vi "frw_array2edf.vi"(6 "channel names":string[](array[string]), 8 "error in":errorcluster, 9 "fs":dbl, 10 "2D array":dbl[][](array[numeric]), 11 "file path":path) -> (0 "error out":errorcluster, 3 "path out":path)   [LabVIEW 2013]
panel:
  out "data_to_write":u16[][](array[numeric])
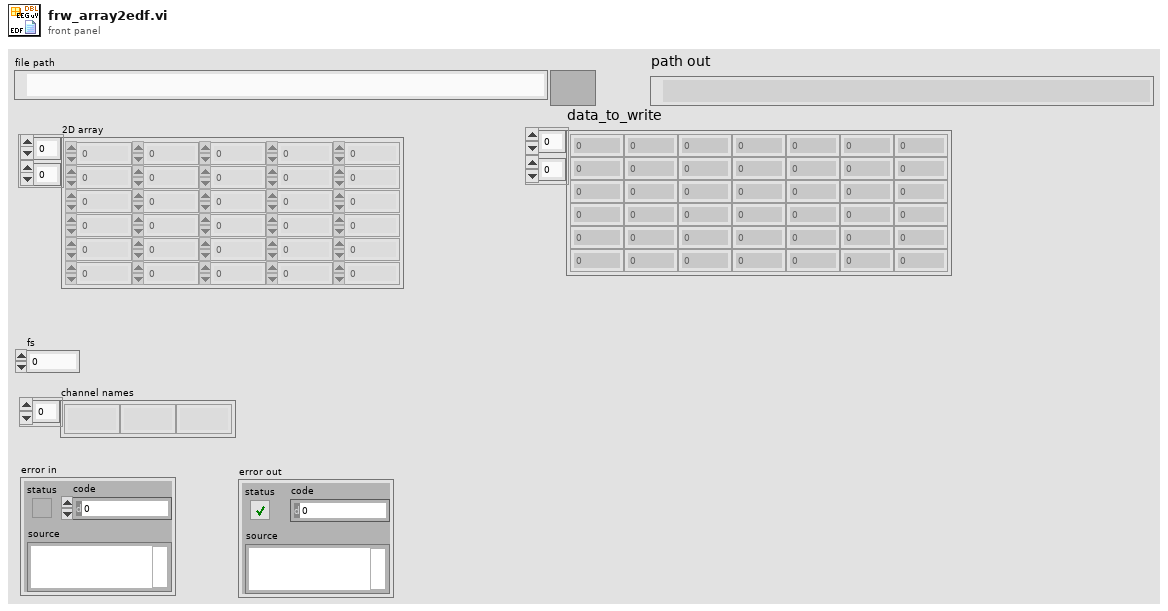
[diagram p1: front panel]
types:
  T1 = enum16{"big-endian, network order", "native, host order", "little-endian"}
  T2 = enum16{"open", "replace", "create", "open or create", "replace or create", "replace or create with confirmation"}
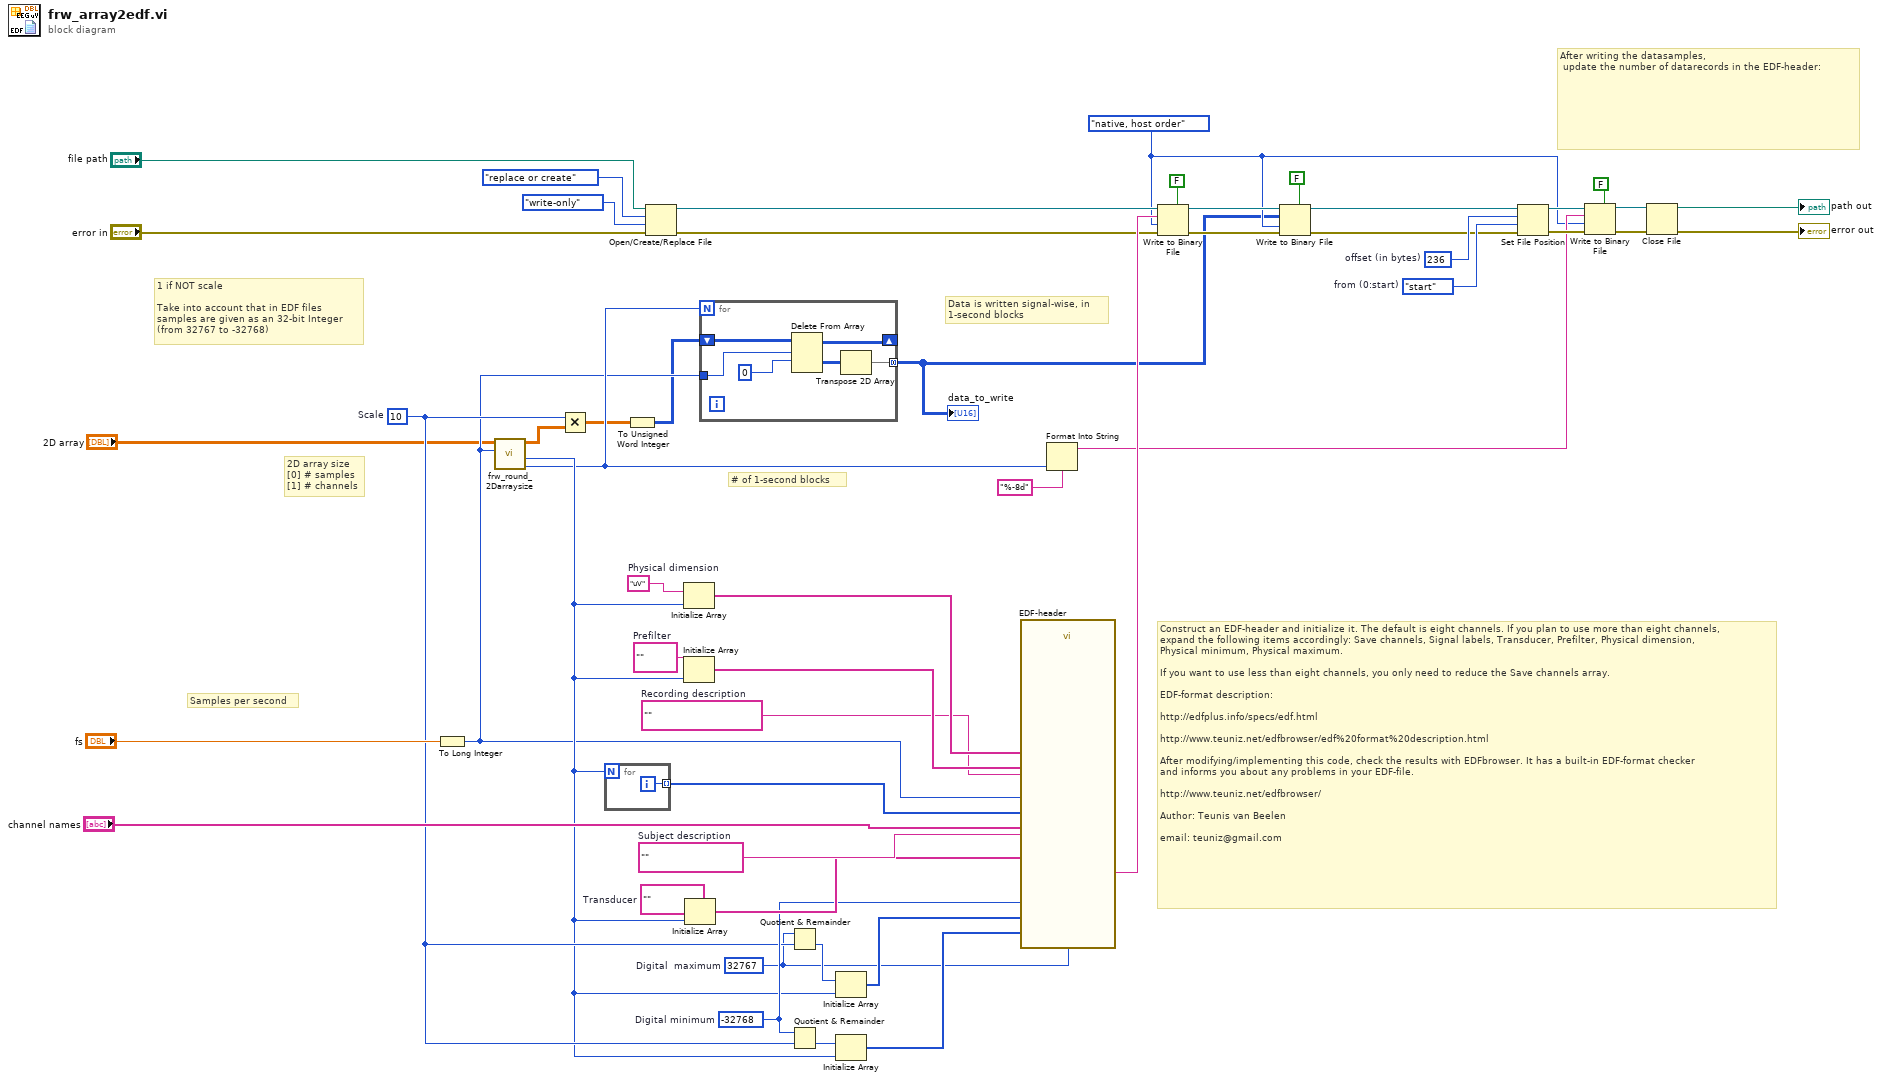
[diagram p0: block diagram]
diagram:
  w15 = 10  # Scale
  w22 = ""  # Transducer
  w23 = ""  # Subject description
  w27 = ""  # Recording description
  w29 = ""  # Prefilter
  w31 = "uV"  # Physical dimension
  w38 = i64 236  # offset (in bytes)
  w39 = enum16{"start", "end", "current"}."start"  # from (0:start)
  w9 = 32767  # Digital  maximum
  w16 = -32768  # Digital minimum
  w12 = T1."native, host order" ("byte order (0:big-endian, network order)")
  # "Data is written signal-wise, in \n1-second blocks"
  # "# of 1-second blocks"
  # "Samples per second"
  # "2D array size\n[0] # samples\n[1] # channels"
  # "1 if NOT scale\n\nTake into account that in EDF files\nsamples are given as an 32-bit Integer\n(from 32767 to -32768)"
  # "After writing the datasamples,\n update the number of datarecords in the EDF-header:"
  # "Construct an EDF-header and initialize it. The default is eight channels. If you plan to use more than eight channels,\nexpand the following items accordingly: Save channels, Signal labels, Transducer, Prefilter, Physical dimension,\nPhysical minimum, Physical maximum.\n\nIf you want to use less than eight channels, you only need to reduce the Save channels array.\n\nEDF-format description:\n\nhttp://edfplus.info/specs/edf.html\n\nhttp://www.teuniz.net/edfbrowser/edf%20format%20description.html\n\nAfter modifying/implementing this code, check the results with EDFbrowser. It has a built-in EDF-format checker\nand informs you about any problems in your EDF-file.\n\nhttp://www.teuniz.net/edfbrowser/\n\nAuthor: Teunis van Beelen\n\nemail: teuniz@gmail.com"
  n1 = To Long Integer(number="fs") -> (32bit integer=w5:i32)
  n2 = call "frw_round_2Darraysize.vi"("block size"=w5, "array in"="2D array") -> ("nBlocks"=w8:i32, "nCol"=w10:i32, "array out"=w7:dbl[][])  [unwired: 6 in, 1 out]
  n3 = Multiply(x=w15, y=w7) -> (x*y=w6:dbl[][])
  n4 = for {
    N: w10 -> [_]
    tunnel: [w52] -> w25 mode=indexing
    i -> [w52]
  }
  n5 = To Unsigned Word Integer(number=w6) -> (unsigned 16bit integer=w4:u16[][])
  n6 = Open/Create/Replace File(file path (use dialog)="file path", error in="error in", operation (0:open)=T2."replace or create", access (0:read/write)=enum16{"read/write", "read-only", "write-only"}."write-only") -> (refnum out=w49:refnum<file>, error out=w14:errorcluster)  [unwired: 2 in, 1 out]
  n7 = Initialize Array(w31, w10) -> (w30:string[])
  n8 = Initialize Array(w29, w10) -> (w28:string[])
  n9 = Initialize Array(w22, w10) -> (w21:string[])
  n10 = for {
    N: w8 -> [_]
    tunnel: w5 -> [w57]
    shift-right: [w55] -> _
    shift-left: w4 -> [w58]
    tunnel: [w53] -> w3 mode=concatenating
    n11 = Delete From Array(array=w58, length=w57, index (row)=0) -> (deleted portion=w54:u16[][], array with subset deleted=w55:u16[][])  [unwired: 1 in]
    n12 = Transpose 2D Array(2D array=w54) -> (transposed array=w53:u16[][])
  }
  "data_to_write" <- w3
  n13 = Quotient & Remainder(x=w9, y=w15) -> (floor(x/y)=w18:i32)  [unwired: 1 out]
  n14 = Quotient & Remainder(x=w16, y=w15) -> (floor(x/y)=w17:i32)  [unwired: 1 out]
  n15 = Initialize Array(w18, w10) -> (w20:i32[])
  n16 = Initialize Array(w17, w10) -> (w19:i32[])
  n17 = call "EDF-header.vi"("Save channels"=w25, "Physical minimum"=w19, "Physical maximum"=w20, "Physical dimension"=w30, "Signal labels"="channel names", "Sample frequency"=w5, "Transducer"=w21, "Subject description"=w23, "Prefilter"=w28, "Digital minimum"=w16, "Digital maximum"=w9, "Recording description"=w27) -> ("EDF-header"=w45:string)  [unwired: 3 in]
  n18 = Format Into String(format string="%-8d", w8) -> (resulting string=w36:string)  [unwired: 2 in, 1 out]
  n19 = Write to Binary File(file (use dialog)=w49, data=w45, error in=w14, 5:FALSE ("prepend array or string size? (T)"), 9:w12) -> (refnum out=w48:refnum<file>, error out=w13:errorcluster)  [unwired: 1 in, 1 out]
  n20 = Write to Binary File(file (use dialog)=w48, data=w3, error in=w13, 5:FALSE ("prepend array or string size? (T)"), 9:w12) -> (refnum out=w37:refnum<file>, error out=w35:errorcluster)  [unwired: 1 in, 1 out]
  n21 = Set File Position(offset (in bytes) (0)=w38, refnum=w37, from (0:start)=w39, error in=w35) -> (refnum out=w43:refnum<file>, error out=w42:errorcluster)
  n22 = Write to Binary File(file (use dialog)=w43, data=w36, error in=w42, 5:FALSE ("prepend array or string size? (T)"), 9:w12) -> (refnum out=w46:refnum<file>, error out=w44:errorcluster)  [unwired: 1 in, 1 out]
  n23 = Close File(refnum=w46, error in=w44) -> (path=→"path out":path, error out=→"error out":errorcluster)
